vi "Stop.vi"(8 "error in":errorcluster, 11 "Virtual Thermometer from CSV in":refnum<class "Virtual Sensor from CSV.lvclass">) -> (0 "error out":errorcluster, 3 "Virtual Thermometer from CSV out":refnum<class "Virtual Sensor from CSV.lvclass">)   [LabVIEW 2024, in "Virtual Sensor from CSV.lvclass"]
uses:
  Virtual Sensor from CSV.lvclass
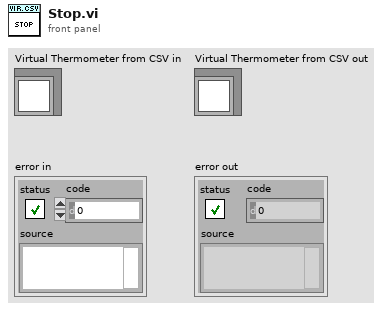
[diagram p1: front panel]
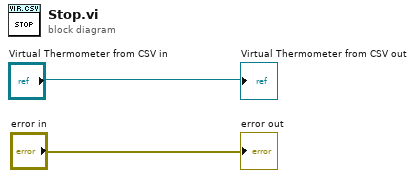
[diagram p0: block diagram]
diagram:
  "error out" <- "error in"
  "Virtual Thermometer from CSV out" <- "Virtual Thermometer from CSV in"
